vi "Actor - SEND - Triggered Event.vi"(7 "Actor Selector":T1, 8 "error in (no error)":errorcluster, 9 "Data":string="Hi!!!", 10 "Events":T2=enum."START Ev") -> (0 "error out":errorcluster)   [LabVIEW 2023, in "Client.lvlib" / "Client.lvclass"]
uses:
  Client.lvclass
  Parent/Parent_Class.lvclass
  Child_1/Child_1_Class.lvclass
  Console/Child_1/Child_2_Class.lvclass
  SW_Interface/Child_3_Class.lvclass
  Message_Distributor/Parent_Class Messages/Parent -  SEND - Triggered Event Msg/Parent -  SEND - Triggered Event Msg.lvclass
  Client - Ctrl - FGV - Action.ctl
  C:/Users/rodri/LabVIEW_Labs/LabVIEW_GitHub/LV-AF-Project/AF_Architecture/Abstraction_Interface_Class/Abstraction_Interface_Class.lvclass
  C:/Program Files (x86)/National Instruments/LabVIEW 2023/vi.lib/ActorFramework/Actor/Actor.lvclass
  C:/Users/rodri/LabVIEW_Labs/LabVIEW_GitHub/LV-AF-Project/AF_Architecture/SW_Interface/Child_3_Class.lvclass
  Child_1/Usr Ev/Child_1 - Ctrl - Enum - Events.ctl
  Client - Ctrl - Actor - Selector.ctl
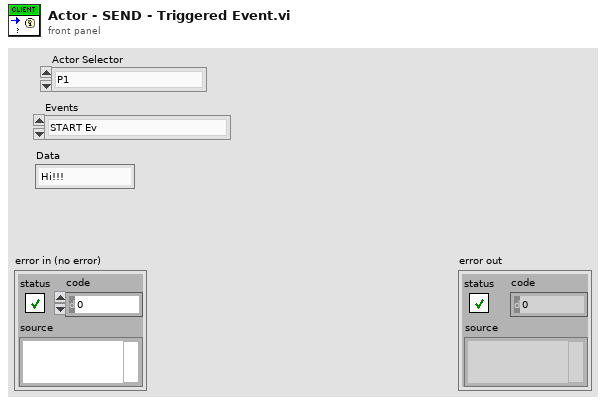
[diagram p1: front panel]
types:
  T1 = typedef "Client.lvlib/Client.lvclass/Client - Ctrl - Actor - Selector.ctl" = enum16{"P1", "C1", "C2", "C3"}
  T2 = typedef "Actor_Child_1.lvlib/Child_1_Class.lvclass/Child_1 - Ctrl - Enum - Events.ctl" = enum16{"SEND MESSAGE Ev", "STOP_ACTOR Ev", "INIT_ACTOR Ev", "START Ev", "STOP Ev", "GET Ev", "SET Ev", "ERROR_HANDLER Ev", "RESET Ev", "T2 Ev", "T3 Ev", "T4 Ev"}
  T3 = typedef "Client.lvlib/Client.lvclass/Client - Ctrl - FGV - Action.ctl" = enum16{"Int", "Get"}
  T4 = map{string, refnum<class "Child_3_Class.lvclass">}
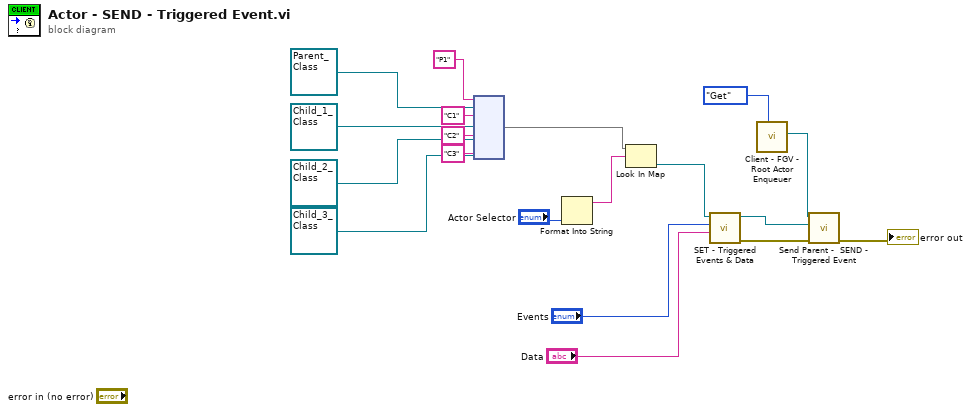
[diagram p0: block diagram]
diagram:
  n1 = node("P1" ("key"), refnum<class "Parent_Class.lvclass"> refnum ("Actor_Parent.lvlib:Parent_Class.lvclass"), "C1" ("key"), refnum<class "Child_1_Class.lvclass"> refnum ("Actor_Child_1.lvlib:Child_1_Class.lvclass"), "C2" ("key"), refnum<class "Child_2_Class.lvclass"> refnum ("Actor_Child_2.lvlib:Child_2_Class.lvclass"), "C3" ("key"), refnum<class "Child_3_Class.lvclass"> refnum ("Actor_Child_3.lvlib:Child_3_Class.lvclass")) -> (w11:T4)
  n2 = Format Into String("Actor Selector") -> (resulting string=w9:string)  [unwired: 3 in, 1 out]
  n3 = Look In Map(map=w11, key=w9) -> (value=w7:refnum<class "Child_3_Class.lvclass">)  [unwired: 1 in, 1 out]
  n4 = call-dynamic "SET - Triggered Events & Data.vi"("Data"="Data", "Events"="Events", "Interface_Class in"=w7) -> ("error out"=w4:errorcluster, "Interface_Class out"=w3:refnum<class "Interface_Class.lvclass">)  [unwired: 7 in]
  n5 = call "Client - FGV - Root Actor Enqueuer.vi"("Action"=Client_-_Ctrl_-_FGV_-_Action."Get") -> ("Root Enqueuer"=w8:refnum<class "Message Enqueuer.lvclass">)  [unwired: 9 in, 1 out]
  n6 = call "Send Parent -  SEND - Triggered Event.vi"("error in (no error)"=w4, "Actor_Interface.lvlib:Interface_Class.lvclass"=w3, "Message Enqueuer"=w8) -> ("error out"=→"error out":errorcluster)  [unwired: 7 in, 1 out]
